vi "Teleop.vi"(10 "Match Info":T2={"Autonomous Elapsed Seconds"=0.0, "TeleOp Elapsed Seconds"=0.0, "Disabled Elapsed Seconds"=0.0, "Visited Autonomous"=FALSE, "Visited TeleOp"=FALSE, "Visited Disabled"=FALSE, "Autonomous Settings"={"Autonomous Style"=enum."Independent", "VI Refnum"=refnum}}, 11 "Call Context":T3) -> ()   [LabVIEW 2015]
doc: "This VI is called for each TeleOp packet received from the DS where the robot is not disabled. It is often used to read from the joysticks and update I/O or to update setpoints for timed control loops. It should complete and return within 20 milliseconds or it may miss DS packets."
uses:
  <vilib>/Rock Robotics/WPI/DriverStation/WPI_DriverStationDerivedRobotMode.ctl
  <vilib>/Rock Robotics/WPI/DriverStation/WPI_DriverStationMatch Info.ctl
  <vilib>/Rock Robotics/WPI/Utilities/WPI_GetSetVariantRefNum.vi
  <vilib>/Rock Robotics/Network Tables/NT Write Boolean Array.vi
  <vilib>/Rock Robotics/Network Tables/NT Write Numeric Array.vi
  <vilib>/Rock Robotics/Network Tables/NT Read Boolean.vi
  <vilib>/Rock Robotics/Network Tables/NT Read Number.vi
  Robot Global Data.vi
  <vilib>/Rock Robotics/WPI/RobotDrive/WPI_RobotDriveArcadeDrive_Standard(NoSaturation).vi
panel:
  out "Ladder Up Start Time":u32
  in  "LadderStateMachine":i32
  out "Accelerations":T1
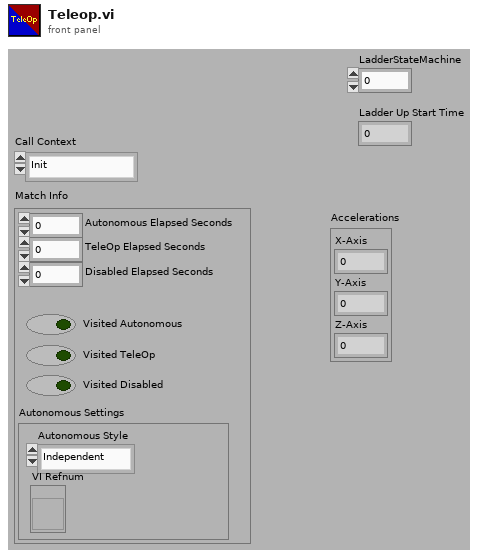
[diagram p1: front panel]
types:
  T1 = cluster{"X-Axis":dbl, "Y-Axis":dbl, "Z-Axis":dbl}
  T2 = typedef "WPI_DriverStationMatch Info.ctl" = cluster{"Autonomous Elapsed Seconds":dbl, "TeleOp Elapsed Seconds":dbl, "Disabled Elapsed Seconds":dbl, "Visited Autonomous":bool, "Visited TeleOp":bool, "Visited Disabled":bool, "Autonomous Settings":cluster{"Autonomous Style":enum16{"Iterative", "Independent"}, "VI Refnum":refnum<vi>}}
  T3 = typedef "WPI_DriverStationDerivedRobotMode.ctl" = enum16{"Init", "Execute", "Stop"}
  T4 = typedef "WPI_RobotDriveDevRef.ctl" = cluster{"DevStatus":errorcluster, "Motors[]":T5[], "Square Inputs":bool, "Max Output":dbl}
  T5 = typedef "WPI_MotorControlDeviceRef.ctl" = cluster{"DeviceStatus":errorcluster, "Type":T6, "PWM":cluster{"PWM Channel":T7, "DeadBand":T8}, "CAN":cluster{"Device Number":u8, "Control Mode":T9, "Semaphore":T10, "Max Vout":dbl, "TalonSRX Control Mode":T11}, "Invert":bool}
  T6 = typedef "WPI_MotorControlType.ctl" = enum16{"PWM", "CAN", "CANTalonSRX"}
  T7 = typedef "FPGA_DIOPWMChannel.ctl" = enum8{"PWM 0", "PWM 1", "PWM 2", "PWM 3", "PWM 4", "PWM 5", "PWM 6", "PWM 7", "PWM 8", "PWM 9", "PWM MXP 0", "PWM MXP 1", "PWM MXP 2", "PWM MXP 3", "PWM MXP 4", "PWM MXP 5", "PWM MXP 6", "PWM MXP 7", "PWM MXP 8", "PWM MXP 9", "Invalid"}
  T8 = typedef "WPI_PWMDeadband.ctl" = cluster{"Name":string, "maxPositivePwm":i32, "minPositivePwm":i32, "centerPwm":i32, "maxNegativePwm":i32, "minNegativePwm":i32, "angularRange":u16}
  T9 = typedef "WPI_CANJaguar_ControlMode.ctl" = enum8{"Percent VBus", "Current", "Speed", "Position", "Voltage"}
  T10 = typedef "Semaphore RefNum" = refnum<k1>
  T11 = typedef "WPI_CANTalonSRX_APIControlMode.ctl" = enum8{"Percent VBus", "Speed", "Position", "Slave", "Unchanged / Invalid", "Voltage Compensation", "Current", "Motion Profile"}
  T12 = typedef "WPI_JoystickDevRef.ctl" = cluster{"Device":T13}
  T13 = typedef "WPI_JoystickDeviceEnum.ctl" = enum16{"USB 0", "USB 1", "USB 2", "USB 3", "USB 4", "USB 5"}
  T14 = typedef "WPI_DigitalInputDevRef.ctl" = cluster{"DevStatus":errorcluster, "DIO Channel":T15}
  T15 = typedef "FPGA_DIOChannel.ctl" = enum8{"DIO 0", "DIO 1", "DIO 2", "DIO 3", "DIO 4", "DIO 5", "DIO 6", "DIO 7", "DIO 8", "DIO 9", "DIO MXP 0", "DIO MXP 1", "DIO MXP 2", "DIO MXP 3", "DIO MXP 4", "DIO MXP 5", "DIO MXP 6", "DIO MXP 7", "DIO MXP 8", "DIO MXP 9", "DIO MXP 10", "DIO MXP 11", "DIO MXP 12", "DIO MXP 13", "DIO MXP 14", "DIO MXP 15", "Invalid"}
  T16 = typedef "WPI_AccelerometerDevRef.ctl" = cluster{"DevStatus":errorcluster, "Scaling":T17, "Analog Channels":T18, "I2C Bus":T20, "SPI Bus":T21, "Accel Range":T22, "ADXL Axes":T23, "Handle":i32, "Device Address":u8, "Accel Type":enum16{"Analog", "ADXL345 I2C", "ADXL345 SPI", "Internal", "ADXL362 SPI"}}
  T17 = typedef "WPI_AccelerometerScaling.ctl" = cluster{"Gain (VoltsPerG)":dbl, "Center Voltage":dbl}
  T18 = typedef "WPI_AccelerometerAnalogChannels.ctl" = cluster{"X-Axis":T19, "Y-Axis":T19, "Z-Axis":T19}
  T19 = typedef "FPGA_AIChannel.ctl" = enum8{"AI 0", "AI 1", "AI 2", "AI 3", "AI MXP 0", "AI MXP 1", "AI MXP 2", "AI MXP 3", "Invalid"}
  T20 = typedef "i2c_bus.ctl" = enum16{"I2C On-Board", "I2C MXP", "Invalid"}
  T21 = typedef "spi_bus.ctl" = enum16{"SPI On-Board, CS0", "SPI On-Board, CS1", "SPI On-Board, CS2", "SPI On-Board, CS3", "SPI MXP", "Invalid"}
  T22 = typedef "ADXL345 Range.ctl" = u8
  T23 = typedef "WPI_AccelerometerADXL345 Axes.ctl" = cluster{"X-Axis":bool, "Y-Axis":bool, "Z-Axis":bool}
  T24 = typedef "WPI_EncoderDevRef.ctl" = cluster{"DevStatus":errorcluster, "EncoderIndex":T25, "CounterIndex":T26, "DistancePerCount":dbl, "Decoding Type":T27}
  T25 = typedef "FPGA_EncoderIdx.ctl" = enum8{"Enc 0", "Enc 1", "Enc 2", "Enc 3", "Enc 4", "Enc 5", "Enc 6", "Enc 7", "Invalid"}
  T26 = typedef "FPGA_CounterCtrSystemIndex.ctl" = enum8{"Ctr 0", "Ctr 1", "Ctr 2", "Ctr 3", "Ctr 4", "Ctr 5", "Ctr 6", "Ctr 7", "Invalid"}
  T27 = typedef "WPI_EncoderType.ctl" = enum16{"1x", "2x", "4x"}
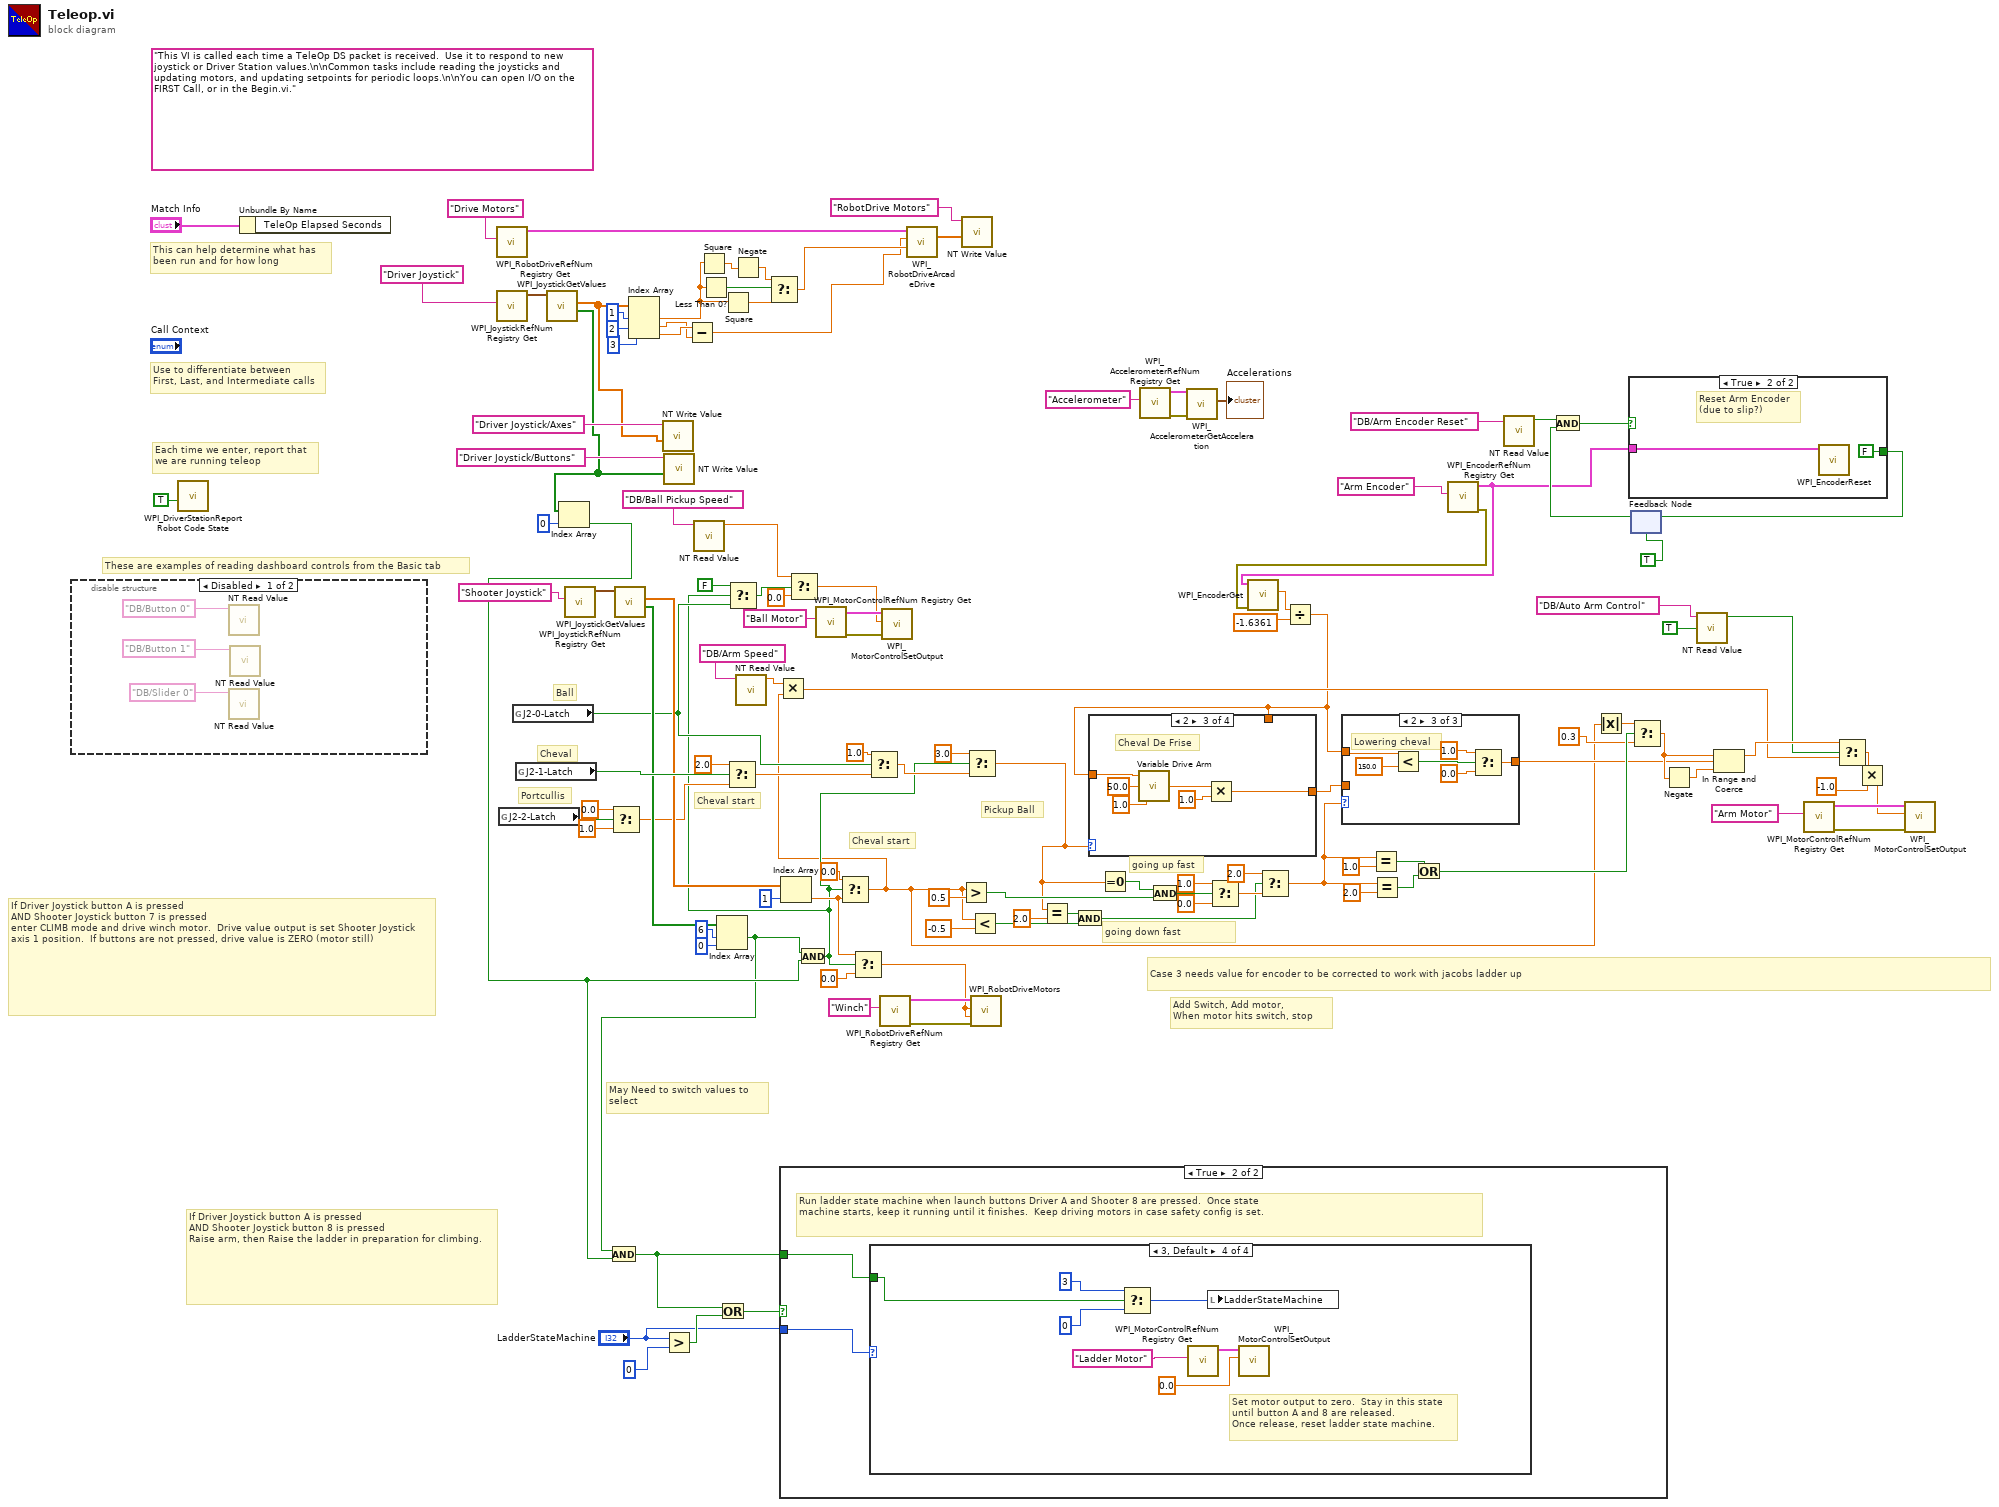
[diagram p0: block diagram]
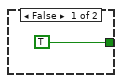
[diagram p2: hidden frame]
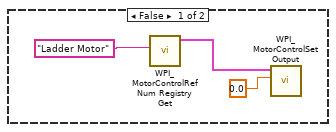
[diagram p4: hidden frame]
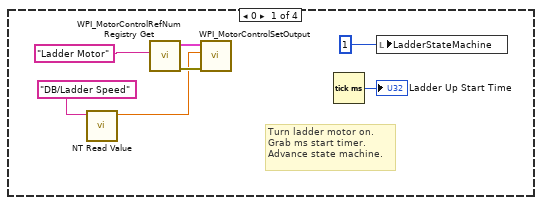
[diagram p5: hidden frame]
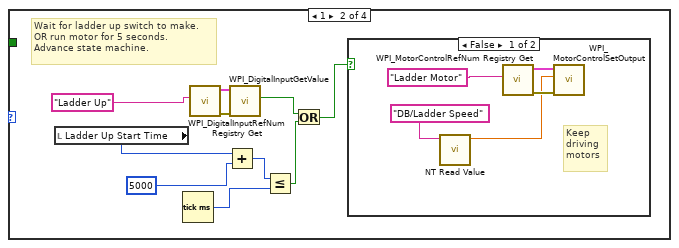
[diagram p6: hidden frame]
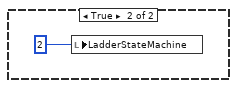
[diagram p7: hidden frame]
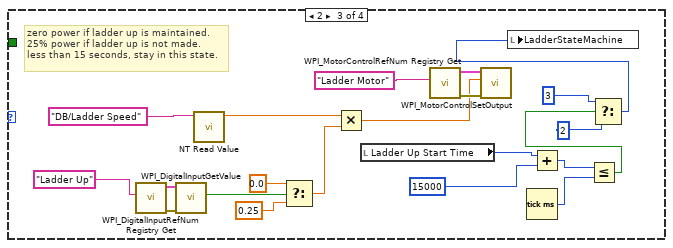
[diagram p8: hidden frame]
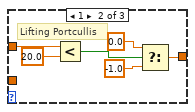
[diagram p10: hidden frame]
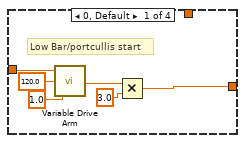
[diagram p11: hidden frame]
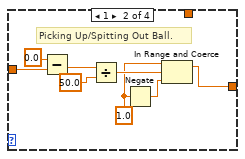
[diagram p12: hidden frame]
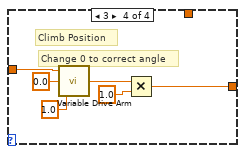
[diagram p13: hidden frame]
diagram:
  (unwired) "This VI is called each time a TeleOp DS packet is received.  Use it to respond to new joystick or Driver Station values.\n\nCommon tasks include reading the joysticks and updating motors, and updating setpoints for periodic loops.\n\nYou can open I/O on the FIRST Call, or in the Begin.vi."
  # "going up fast"
  # "going down fast"
  # "If Driver Joystick button A is pressed\nAND Shooter Joystick button 8 is pressed\nRaise arm, then Raise the ladder in preparation for climbing."
  # "If Driver Joystick button A is pressed\nAND Shooter Joystick button 7 is pressed\nenter CLIMB mode and drive winch motor.  Drive value output is set Shooter Joystick axis 1 position.  If buttons are not pressed, drive value is ZERO (motor still)"
  # "Add Switch, Add motor, \nWhen motor hits switch, stop"
  # "Portcullis"
  # "Ball"
  # "Cheval"
  # "May Need to switch values to \nselect"
  # "Case 3 needs value for encoder to be corrected to work with jacobs ladder up"
  # "Cheval start"
  # "Pickup Ball"
  # "Cheval start"
  # "These are examples of reading dashboard controls from the Basic tab"
  # "Each time we enter, report that\nwe are running teleop"
  # "Use to differentiate between\nFirst, Last, and Intermediate calls"
  # "This can help determine what has\nbeen run and for how long"
  n1 = disable-structure shown="Disabled" {
    frame Disabled {
      n2 = call-poly <vilib>:"NT Read Value.vi"("Name"="DB/Button 0" ("refnum name")) -> ("Boolean"=w124:bool)  [unwired: 9 in, 1 out]
      n3 = call-poly <vilib>:"NT Read Value.vi"("Name"="DB/Slider 0" ("refnum name")) -> ("Numeric"=w126:dbl)  [unwired: 9 in, 1 out]
      n4 = call-poly <vilib>:"NT Read Value.vi"("Name"="DB/Button 1" ("refnum name")) -> ("Boolean"=w125:bool)  [unwired: 9 in, 1 out]
    }
    frame Enabled {
    }
  }
  n5 = call <vilib>:"WPI_DriverStationReport Robot Code State.vi"("TeleOp"=TRUE ("Autonomous")) -> ()  [unwired: 10 in, 1 out]
  n6 = Unbundle By Name("Match Info") -> ()  [unwired: 1 out]
  n7 = call <vilib>:"WPI_RobotDriveRefNum Registry Get.vi"("refnum name"="Drive Motors") -> ("RobotDriveDevRef"=w120:T4)  [unwired: 1 in, 9 out]
  n8 = call <vilib>:"WPI_JoystickRefNum Registry Get.vi"("refnum name"="Driver Joystick") -> ("JoystickDevRef"=w118:T12)  [unwired: 1 in, 9 out]
  n9 = global read "Robot Global Data.vi" "J2-2-Latch"() -> (w37:bool)
  n10 = global read "Robot Global Data.vi" "J2-0-Latch"() -> (w33:bool)
  n11 = global read "Robot Global Data.vi" "J2-1-Latch"() -> (w94:bool)
  n12 = call <vilib>:"WPI_JoystickGetValues.vi"("JoystickDevRef"=w118) -> ("Buttons"=w107:bool[], "Axes"=w108:dbl[])  [unwired: 6 in, 3 out]
  n13 = Index Array(array=w107, index=0) -> (element=w30:bool)
  n14 = call <vilib>:"WPI_JoystickRefNum Registry Get.vi"("refnum name"="Shooter Joystick") -> ("JoystickDevRef"=w106:T12)  [unwired: 1 in, 9 out]
  n15 = Select(t=0.0, s=w37, f=1.0) -> (s? t:f=w38:dbl)
  n16 = call <vilib>:"WPI_JoystickGetValues.vi"("JoystickDevRef"=w106) -> ("Buttons"=w76:bool[], "Axes"=w67:dbl[])  [unwired: 6 in, 3 out]
  n17 = Index Array(array=w108, index #1=1 ("index"), index #2=2 ("index"), index #3=3 ("index")) -> (element #1=w63:dbl, element #2=w60:dbl, element #3=w61:dbl)
  n18 = call-poly <vilib>:"NT Write Value.vi"("Numeric Array"=w108, "Name"="Driver Joystick/Axes") -> ()  [unwired: 9 in, 1 out]
  n19 = call-poly <vilib>:"NT Write Value.vi"("Boolean Array"=w107, "Name"="Driver Joystick/Buttons") -> ()  [unwired: 9 in, 1 out]
  n20 = Greater?(x="LadderStateMachine", y=0) -> (0:w12:bool)
  n21 = Subtract(x=w61, y=w60) -> (x-y=w59:dbl)
  n22 = call-poly <vilib>:"NT Read Value.vi"("Name"="DB/Ball Pickup Speed") -> ("Numeric"=w20:dbl)  [unwired: 9 in, 1 out]
  n23 = Square(x=w63) -> (x^2=w112:dbl)
  n24 = Less Than 0?(x=w63) -> (x < 0?=w114:bool)
  n25 = Index Array(array=w76, index #1=6 ("index"), index #2=0 ("index")) -> (element #1=w8:bool)  [unwired: 1 out]
  n26 = And(x=w8, y=w30) -> (x .and. y?=w9:bool)
  n27 = Or(x=w9, y=w12) -> (x .or. y?=w11:bool)
  n28 = Square(x=w63) -> (x^2=w111:dbl)
  n29 = Select(t=2.0, s=w94, f=w38) -> (s? t:f=w95:dbl)
  n30 = Negate(x=w112) -> (-x=w113:dbl)
  n31 = call-poly <vilib>:"NT Read Value.vi"("Name"="DB/Arm Speed") -> ("Numeric"=w23:dbl)  [unwired: 9 in, 1 out]
  n32 = Select(t=w113, s=w114, f=w111) -> (s? t:f=w66:dbl)
  n33 = case shown="True" w11 {
    tunnel: "LadderStateMachine" -> [_ w134]
    tunnel: w9 -> [_ w133]
    frame False {
      n34 = call <vilib>:"WPI_MotorControlRefNum Registry Get.vi"("refnum name"="Ladder Motor") -> ("MotorControlDevRef"=w130:T5)  [unwired: 9 in, 1 out]
      n35 = call <vilib>:"WPI_MotorControlSetOutput.vi"("Output"=0.0, "MotorControlDevRef"=w130) -> ()  [unwired: 7 in, 3 out]
    }
    frame True {
      # "Run ladder state machine when launch buttons Driver A and Shooter 8 are pressed.  Once state\nmachine starts, keep it running until it finishes.  Keep driving motors in case safety config is set."
      n36 = case shown="3, Default" w134 {
        tunnel: w133 -> [_ _ _ w183]
        frame 0 {
          # "Turn ladder motor on.\nGrab ms start timer.\nAdvance state machine."
          n37 = call-poly <vilib>:"NT Read Value.vi"("Name"="DB/Ladder Speed") -> ("Numeric"=w137:dbl)  [unwired: 9 in, 1 out]
          n38 = call <vilib>:"WPI_MotorControlRefNum Registry Get.vi"("refnum name"="Ladder Motor") -> ("error out"=w141:errorcluster, "MotorControlDevRef"=w140:T5)  [unwired: 9 in]
          n39 = call <vilib>:"WPI_MotorControlSetOutput.vi"("error in (no error)"=w141, "Output"=w137, "MotorControlDevRef"=w140) -> ()  [unwired: 6 in, 3 out]
          n40 = Tick Count (ms)() -> (millisecond timer value=→"Ladder Up Start Time":u32)
          n41 = local write "LadderStateMachine"(1 ("LadderStateMachine")) -> ()
        }
        frame 1 {
          # "Wait for ladder up switch to make.\nOR run motor for 5 seconds.\nAdvance state machine."
          n42 = local read "Ladder Up Start Time"() -> (w147:u32)
          n43 = Tick Count (ms)() -> (millisecond timer value=w145:u32)
          n44 = call <vilib>:"WPI_DigitalInputRefNum Registry Get.vi"("refnum name"="Ladder Up") -> ("error out"=w151:errorcluster, "DigitalInputDevRef"=w149:T14)  [unwired: 9 in]
          n45 = Add(x=w147, y=u32 5000) -> (x+y=w146:u32)
          n46 = call <vilib>:"WPI_DigitalInputGetValue.vi"("error in (no error)"=w151, "DigitalInputDevRef"=w149) -> ("Value"=w142:bool)  [unwired: 7 in, 2 out]
          n47 = Less Or Equal?(x=w146, y=w145) -> (x <= y?=w143:bool)
          n48 = Or(x=w142, y=w143) -> (x .or. y?=w144:bool)
          n49 = case shown="False" w144 {
            frame False {
              # "Keep\ndriving \nmotors"
              n50 = call-poly <vilib>:"NT Read Value.vi"("Name"="DB/Ladder Speed") -> ("Numeric"=w152:dbl)  [unwired: 9 in, 1 out]
              n51 = call <vilib>:"WPI_MotorControlRefNum Registry Get.vi"("refnum name"="Ladder Motor") -> ("error out"=w156:errorcluster, "MotorControlDevRef"=w155:T5)  [unwired: 9 in]
              n52 = call <vilib>:"WPI_MotorControlSetOutput.vi"("error in (no error)"=w156, "Output"=w152, "MotorControlDevRef"=w155) -> ()  [unwired: 6 in, 3 out]
            }
            frame True {
              n53 = local write "LadderStateMachine"(2 ("LadderStateMachine")) -> ()
            }
          }
        }
        frame 2 {
          # "zero power if ladder up is maintained.\n25% power if ladder up is not made.\nless than 15 seconds, stay in this state."
          n54 = call <vilib>:"WPI_DigitalInputRefNum Registry Get.vi"("refnum name"="Ladder Up") -> ("error out"=w172:errorcluster, "DigitalInputDevRef"=w170:T14)  [unwired: 9 in]
          n55 = call <vilib>:"WPI_DigitalInputGetValue.vi"("error in (no error)"=w172, "DigitalInputDevRef"=w170) -> ("Value"=w169:bool)  [unwired: 7 in, 2 out]
          n56 = call-poly <vilib>:"NT Read Value.vi"("Name"="DB/Ladder Speed") -> ("Numeric"=w174:dbl)  [unwired: 9 in, 1 out]
          n57 = Select(t=0.0, s=w169, f=0.25 ("y")) -> (s? t:f=w166:dbl)
          n58 = Multiply(x=w174, y=w166) -> (x*y=w173:dbl)
          n59 = local read "Ladder Up Start Time"() -> (w164:u32)
          n60 = call <vilib>:"WPI_MotorControlRefNum Registry Get.vi"("refnum name"="Ladder Motor") -> ("error out"=w178:errorcluster, "MotorControlDevRef"=w177:T5)  [unwired: 9 in]
          n61 = call <vilib>:"WPI_MotorControlSetOutput.vi"("error in (no error)"=w178, "Output"=w173, "MotorControlDevRef"=w177) -> ()  [unwired: 6 in, 3 out]
          n62 = Tick Count (ms)() -> (millisecond timer value=w162:u32)
          n63 = Add(x=w164, y=u32 15000) -> (x+y=w163:u32)
          n64 = Less Or Equal?(x=w163, y=w162) -> (x <= y?=w161:bool)
          n65 = Select(t=3 ("LadderStateMachine"), s=w161, f=2) -> (s? t:f=w158:i32)
          n66 = local write "LadderStateMachine"(w158) -> ()
        }
        frame 3, Default {
          # "Set motor output to zero.  Stay in this state\nuntil button A and 8 are released.\nOnce release, reset ladder state machine."
          n67 = Select(t=3 ("y"), s=w183, f=0 ("y")) -> (s? t:f=w182:i32)
          n68 = call <vilib>:"WPI_MotorControlRefNum Registry Get.vi"("refnum name"="Ladder Motor") -> ("MotorControlDevRef"=w181:T5)  [unwired: 9 in, 1 out]
          n69 = local write "LadderStateMachine"(w182) -> ()
          n70 = call <vilib>:"WPI_MotorControlSetOutput.vi"("Output"=0.0, "MotorControlDevRef"=w181) -> ()  [unwired: 7 in, 3 out]
        }
      }
    }
  }
  n71 = Index Array(array=w67, index=1) -> (element=w58:dbl)
  n72 = And(x=w8, y=w30) -> (x .and. y?=w31:bool)
  n73 = Select(t=FALSE, s=w31, f=w33) -> (s? t:f=w34:bool)
  n74 = Select(t=w20, s=w34, f=0.0) -> (s? t:f=w98:dbl)
  n75 = call <vilib>:"WPI_MotorControlRefNum Registry Get.vi"("refnum name"="Ball Motor") -> ("error out"=w99:errorcluster, "MotorControlDevRef"=w100:T5)  [unwired: 9 in]
  n76 = Select(t=0.0, s=w31, f=w58) -> (s? t:f=w24:dbl)
  n77 = Multiply(x=w23, y=w24) -> (x*y=w18:dbl)
  n78 = Select(t=w58, s=w31, f=0.0) -> (s? t:f=w73:dbl)
  n79 = Select(t=1.0, s=w33, f=w95) -> (s? t:f=w42:dbl)
  n80 = call <vilib>:"WPI_RobotDriveRefNum Registry Get.vi"("refnum name"="Winch") -> ("error out"=w75:errorcluster, "RobotDriveDevRef"=w74:T4)  [unwired: 9 in]
  n81 = call <vilib>:"WPI_MotorControlSetOutput.vi"("error in (no error)"=w99, "Output"=w98, "MotorControlDevRef"=w100) -> ()  [unwired: 6 in, 3 out]
  n82 = call-poly <vilib>:"WPI_RobotDriveArcadeDrive.vi"("Y axis value"=w66, "X axis value"=w59, "RobotDriveDevRef"=w120) -> ("Motor Values"=w117:dbl[])  [unwired: 6 in, 2 out]
  n83 = Greater?(x=w24, y=0.5) -> (0:w90:bool)
  n84 = call-poly <vilib>:"NT Write Value.vi"("Numeric Array"=w117, "Name"="RobotDrive Motors") -> ()  [unwired: 9 in, 1 out]
  n85 = Select(t=3.0, s=w31, f=w42) -> (s? t:f=w43:dbl)
  n86 = Less?(x=w24, y=-0.5) -> (x < y?=w84:bool)
  n87 = call <vilib>:"WPI_RobotDriveMotors.vi"("error in (no error)"=w75, "RightSpeed"=w73, "LeftSpeed"=w73, "RobotDriveDevRef"=w74) -> ()  [unwired: 5 in, 3 out]
  n88 = Equal?(x=w43, y=2.0) -> (x = y?=w83:bool)
  n89 = And(x=w83, y=w84) -> (x .and. y?=w80:bool)
  n90 = Equal To 0?(x=w43) -> (x = 0?=w93:bool)
  n91 = call <vilib>:"WPI_AccelerometerRefNum Registry Get.vi"("refnum name"="Accelerometer") -> ("error out"=w70:errorcluster, "AccelerometerDevRef"=w69:T16)  [unwired: 9 in]
  n92 = And(x=w93, y=w90) -> (x .and. y?=w89:bool)
  n93 = call <vilib>:"WPI_AccelerometerGetAcceleration.vi"("error in"=w70, "AccelerometerDevRef"=w69) -> ("Accelerations"=→"Accelerations":T1)  [unwired: 7 in, 2 out]
  n94 = Select(t=1.0, s=w89, f=0.0) -> (s? t:f=w81:dbl)
  n95 = Select(t=2.0, s=w80, f=w81) -> (s? t:f=w55:dbl)
  n96 = Equal?(x=w55, y=1.0) -> (x = y?=w53:bool)
  n97 = Equal?(x=w55, y=2.0) -> (x = y?=w52:bool)
  n98 = Or(x=w53, y=w52) -> (x .or. y?=w51:bool)
  n99 = call <vilib>:"WPI_EncoderRefNum Registry Get.vi"("refnum name"="Arm Encoder") -> ("error out"=w5:errorcluster, "EncoderDevRef"=w6:T24)  [unwired: 9 in]
  n100 = call <vilib>:"WPI_EncoderGet.vi"("error in (no error)"=w5, "EncoderDevRef"=w6) -> ("Distance"=w3:dbl)  [unwired: 4 in, 5 out]
  n101 = Divide(x=w3, y=-1.6361 ("Arm Calibration")) -> (x/y=w2:dbl)
  n102 = case shown="2" w43 {
    tunnel: w2 -> [w191 w194 w200 w206]
    tunnel: [w188 w192 w201 w207] -> w86
    tunnel: w2 -> [_ _ _ _]
    frame 0, Default {
      # "Low Bar/portcullis start"
      n103 = call "Variable Drive Arm.vi"("Max Speed"=1.0, "Wanted Angle"=120.0, "Encoder"=w191) -> ("Motor Controller"=w187:dbl)
      n104 = Multiply(x=w187, y=3.0) -> (x*y=w188:dbl)
    }
    frame 1 {
      w196 = 1.0 ("Max Speed")
      # "Picking Up/Spitting Out Ball."
      n105 = Subtract(x=0.0 ("Wanted Angle"), y=w194) -> (x-y=w199:dbl)
      n106 = Divide(x=w199, y=50.0) -> (x/y=w198:dbl)
      n107 = Negate(x=w196) -> (-x=w197:dbl)
      n108 = In Range and Coerce(upper limit=w196, x=w198, lower limit=w197) -> (coerced(x)=w192:dbl)  [unwired: 1 out]
    }
    frame 2 {
      # "Cheval De Frise"
      n109 = call "Variable Drive Arm.vi"("Max Speed"=1.0, "Wanted Angle"=50.0, "Encoder"=w200) -> ("Motor Controller"=w203:dbl)
      n110 = Multiply(x=w203, y=1.0) -> (x*y=w201:dbl)
    }
    frame 3 {
      # "Change 0 to correct angle"
      # "Climb Position"
      n111 = call "Variable Drive Arm.vi"("Max Speed"=1.0, "Wanted Angle"=0.0, "Encoder"=w206) -> ("Motor Controller"=w209:dbl)
      n112 = Multiply(x=w209, y=1.0) -> (x*y=w207:dbl)
    }
  }
  n113 = case shown="2" w55 {
    tunnel: w2 -> [_ w215 w221]
    tunnel: [w212 w213 w219] -> w46
    tunnel: w86 -> [w212 _ _]
    frame 0, Default {
    }
    frame 1 {
      # "Lifting Portcullis"
      n114 = Less?(x=w215, y=20.0) -> (x < y?=w216:bool)
      n115 = Select(t=0.0, s=w216, f=-1.0) -> (s? t:f=w213:dbl)
    }
    frame 2 {
      # "Lowering cheval"
      n116 = Less?(x=w221, y=150.0) -> (x < y?=w222:bool)
      n117 = Select(t=1.0, s=w222, f=0.0) -> (s? t:f=w219:dbl)
    }
  }
  n118 = call-poly <vilib>:"NT Read Value.vi"("Name"="DB/Arm Encoder Reset") -> ("Boolean"=w17:bool)  [unwired: 9 in, 1 out]
  n119 = Absolute Value(x=w24) -> (abs(x)=w50:dbl)
  n120 = feedback #1(TRUE) -> (w15:bool)
  n121 = And(x=w17, y=w15) -> (x .and. y?=w1:bool)
  n122 = case shown="True" w1 {
    tunnel: [TRUE FALSE] -> w14
    tunnel: w6 -> [_ w226]
    frame False {
    }
    frame True {
      # "Reset Arm Encoder\n(due to slip?)"
      n123 = call <vilib>:"WPI_EncoderReset.vi"("EncoderDevRef"=w226) -> ()  [unwired: 9 in, 2 out]
    }
  }
  n124 = feedback-in #1(w14) -> ()
  n125 = Select(t=w50, s=w51, f=0.3) -> (s? t:f=w47:dbl)
  n126 = Negate(x=w47) -> (-x=w48:dbl)
  n127 = call-poly <vilib>:"NT Read Value.vi"("Default Value"=TRUE, "Name"="DB/Auto Arm Control") -> ("Boolean"=w25:bool)  [unwired: 8 in, 1 out]
  n128 = In Range and Coerce(upper limit=w47, x=w46, lower limit=w48) -> (coerced(x)=w49:dbl)  [unwired: 1 out]
  n129 = call <vilib>:"WPI_MotorControlRefNum Registry Get.vi"("refnum name"="Arm Motor") -> ("error out"=w102:errorcluster, "MotorControlDevRef"=w103:T5)  [unwired: 9 in]
  n130 = Select(t=w49, s=w25, f=w18) -> (s? t:f=w57:dbl)
  n131 = Multiply(x=w57, y=-1.0) -> (x*y=w29:dbl)
  n132 = call <vilib>:"WPI_MotorControlSetOutput.vi"("error in (no error)"=w102, "Output"=w29, "MotorControlDevRef"=w103) -> ()  [unwired: 6 in, 3 out]
